vi "FGGA_files_transfer.vi"(0 "Flight_num":string, 1 "Get current?":bool, 5 "Date":string, 7 "Flight Folder Path":path) -> (15 "error IO":errorcluster)   [LabVIEW 2014]
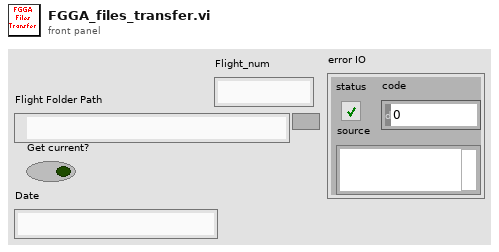
[diagram p1: front panel]
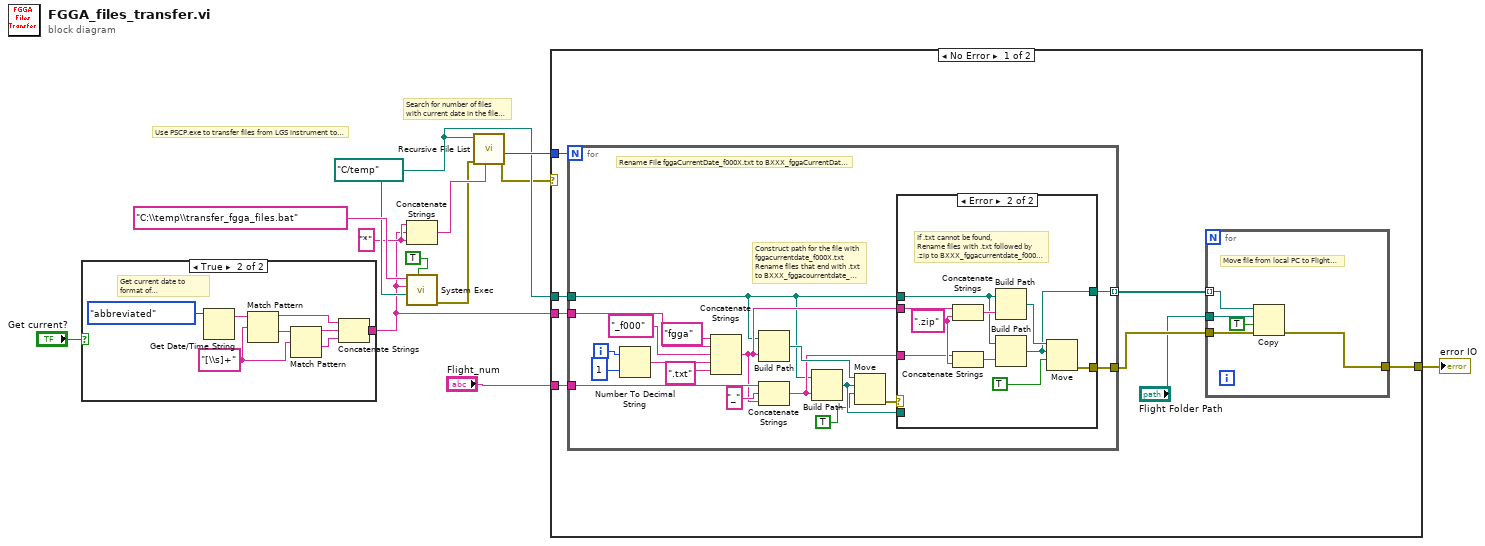
[diagram p0: block diagram]
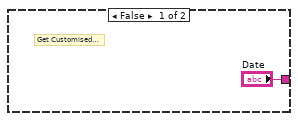
[diagram p2: hidden frame]
diagram:
  w8 = "*"
  w9 = path "C:/temp" ("working directory")
  # "Search for number of files\nwith current date in the file name"
  # "Use PSCP.exe to transfer files from LGS instrument to Local PC"
  n1 = case shown="True" "Get current?" {
    tunnel: ["Date" w14] -> w6
    frame False {
      # "Get Customised Date"
    }
    frame True {
      w19 = "[\\s]+" ("regular expression")
      # "Get current date to format of\n01Jan11 for example"
      n2 = Get Date/Time String(date format (0)=enum16{"short", "long", "abbreviated"}."abbreviated") -> (date string=w20:string)  [unwired: 2 in, 1 out]
      n3 = Match Pattern(string=w20, regular expression=w19) -> (before substring=w17:string, after substring=w18:string)  [unwired: 1 in, 2 out]
      n4 = Match Pattern(string=w18, regular expression=w19) -> (before substring=w16:string, after substring=w15:string)  [unwired: 1 in, 2 out]
      n5 = Concatenate Strings(w17, w16, w15) -> (w14:string)
    }
  }
  n6 = Concatenate Strings(w8, w6, w8) -> (w7:string)
  n7 = call <vilib>:"System Exec.vi"("wait until completion? (T)"=TRUE, "working directory"=w9, "standard input"=w6, "command line"="C:\\temp\\transfer_fgga_files.bat") -> ("error out"=w3:errorcluster)  [unwired: 4 in, 3 out]
  n8 = call <vilib>:"Recursive File List.vi"("pattern"=w7, "error in (no error)"=w3, "Folder Path"=w9) -> ("error out"=w2:errorcluster, "Number of Files"=w12:i32)  [unwired: 4 in, 3 out]
  n9 = case shown="No Error" w2 {
    selector: w2 -> [_ w65]
    tunnel: w12 -> [w29 _]
    tunnel: w9 -> [w28 _]
    tunnel: w6 -> [w27 _]
    tunnel: [w26 w65] -> w5
    tunnel: "Flight_num" -> [w25 _]
    frame No Error {
      n10 = for {
        N: w29 -> [_]
        tunnel: w28 -> [w35]
        tunnel: w27 -> [w47]
        tunnel: w25 -> [w46]
        tunnel: [w39] -> w23
        tunnel: [w38] -> w24 mode=indexing
        i -> [w52]
        # "Rename File fggaCurrentDate_f000X.txt to BXXX_fggaCurrentDate_f000X.txt"
        # "Construct path for the file with\nfggacurrentdate_f000X.txt\nRename files that end with .txt\nto BXXX_fggacourrentdate_f000X.txt"
        n11 = Number To Decimal String(number=w52, width (-)=i16 1) -> (decimal integer string=w51:string)
        n12 = Concatenate Strings("fgga" ("name or relative path"), w47, "_f000" ("string"), w51, ".txt" ("string")) -> (w41:string)
        n13 = Build Path(base path=w35, name or relative path=w41) -> (appended path=w43:path)
        n14 = Concatenate Strings(w46, "_" ("string"), w41) -> (w40:string)
        n15 = Build Path(base path=w35, name or relative path=w40) -> (appended path=w37:path)
        n16 = Move(source path=w43, 9:TRUE ("overwrite (F)"), 10:w37) -> (error out=w42:errorcluster)  [unwired: 2 in, 2 out]
        n17 = case shown="Error" w42 {
          selector: w42 -> [w54 _]
          tunnel: w41 -> [_ w64]
          tunnel: w40 -> [_ w60]
          tunnel: [w54 w58] -> w39
          tunnel: [w53 w57] -> w38
          tunnel: w37 -> [w53 _]
          tunnel: w35 -> [_ w55]
          frame No Error {
          }
          frame Error {
            w61 = ".zip" ("string")
            # "If .txt cannot be found,\nRename files with .txt followed by\n.zip to BXXX_fggacurrentdate_f000X.txt.zip"
            n18 = Concatenate Strings(w64, w61) -> (w63:string)
            n19 = Concatenate Strings(w60, w61) -> (w59:string)
            n20 = Build Path(base path=w55, name or relative path=w63) -> (appended path=w62:path)
            n21 = Build Path(base path=w55, name or relative path=w59) -> (appended path=w57:path)
            n22 = Move(source path=w62, 9:TRUE ("overwrite (F)"), 10:w57) -> (error out=w58:errorcluster)  [unwired: 2 in, 2 out]
          }
        }
      }
      n23 = for {
        tunnel: w24 -> [w34] mode=indexing
        tunnel: w23 -> [w33]
        tunnel: "Flight Folder Path" -> [w32]
        tunnel: [w31] -> w26
        # "Move file from local PC to Flight Folder"
        n24 = Copy(8:w33, 9:TRUE ("overwrite (F)"), 10:w32, 11:w34) -> (0:w31:errorcluster)  [unwired: 1 in, 2 out]
      }
    }
    frame Error {
    }
  }
  "error IO" <- w5
